vi "Login.vi"() -> (3 "Username":string)   [LabVIEW 2018]
panel:
  out "Password":bool
  in  "Password:":string
  in  "OK Button":bool
  in  "Username:":enum16{"Operator", "Administrator"}(ring)
  # "Log in"
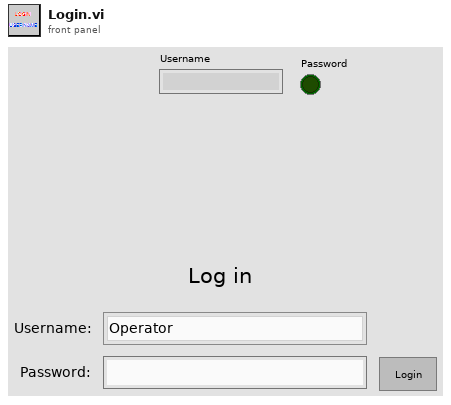
[diagram p1: front panel]
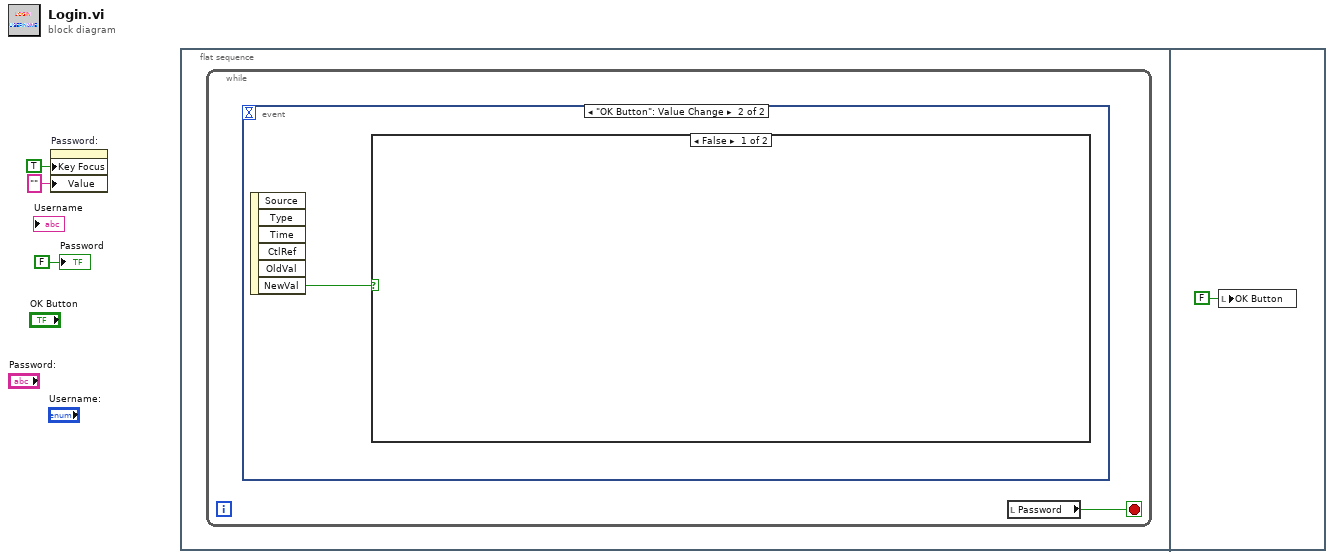
[diagram p0: block diagram]
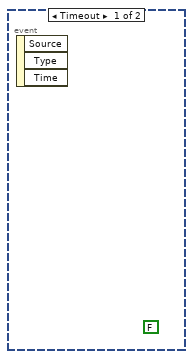
[diagram p2: hidden frame]
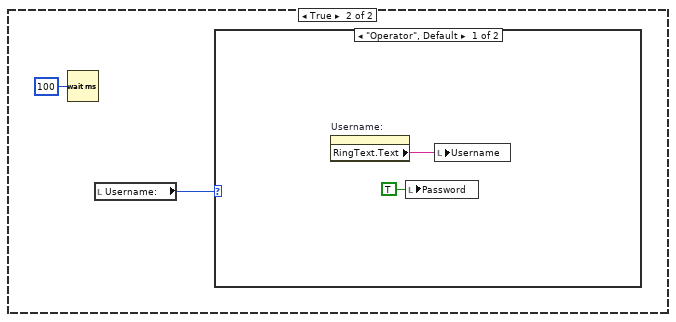
[diagram p3: hidden frame]
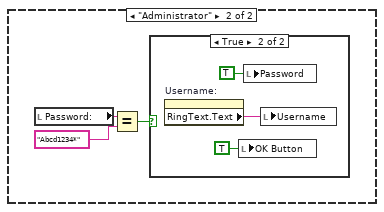
[diagram p4: hidden frame]
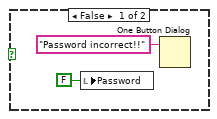
[diagram p5: hidden frame]
diagram:
  n1 = property on="Password:" class="Str"("Key Focus"=TRUE, "Value"="" ("Password:")) -> ()  [unwired: 2 in, 2 out]
  n2 = flat-sequence {
    frame #0 {
      n3 = while {
        stop <- w4 stop-if-true
        n4 = event shown="[1] \"OK Button\": Value Change" {
          selector: _ -> [_ _]
          dyn-events: _ -> [_ _]
          timeout: _ -> [_ _]
          event Timeout {
            (unwired) FALSE
            n5 = event-data() -> ()  [unwired: 1 in, 3 out]
          }
          event "OK Button": Value Change {
            n6 = event-data() -> ("NewVal"=w5:bool)  [unwired: 1 in, 5 out]
            n7 = case shown="False" w5 {
              frame False {
              }
              frame True {
                n8 = Wait (ms)(milliseconds to wait=u32 100) -> ()  [unwired: 1 out]
                n9 = local read "Username:"() -> (w6:enum16{"Operator", "Administrator"})
                n10 = case shown="\"Operator\", Default" w6 {
                  frame "Operator", Default {
                    n11 = property on="Username:" class="Enum (strict)"() -> ("RingText.Text"=w8:string)  [unwired: 2 in, 2 out]
                    n12 = local write "Password"(TRUE ("Password")) -> ()
                    n13 = local write "Username"(w8) -> ()
                  }
                  frame "Administrator" {
                    n14 = local read "Password:"() -> (w10:string)
                    n15 = Equal?(x=w10, y="Abcd1234*") -> (x = y?=w11:bool)
                    n16 = case shown="True" w11 {
                      frame False {
                        n17 = local write "Password"(FALSE ("Password")) -> ()
                        n18 = One Button Dialog(message="Password incorrect!!") -> ()  [unwired: 1 in, 1 out]
                      }
                      frame True {
                        n19 = property on="Username:" class="Enum (strict)"() -> ("RingText.Text"=w15:string)  [unwired: 2 in, 2 out]
                        n20 = local write "OK Button"(TRUE ("OK Button")) -> ()
                        n21 = local write "Password"(TRUE ("Password")) -> ()
                        n22 = local write "Username"(w15) -> ()
                      }
                    }
                  }
                }
              }
            }
          }
        }
        n23 = local read "Password"() -> (w4:bool)
      }
    }
    frame #1 {
      n24 = local write "OK Button"(FALSE ("OK Button")) -> ()
    }
  }
  "Password" <- FALSE ("Password")
